vi "Set Emergency.vi"(8 "error in (no error)":errorcluster, 10 "Emergency":bool=TRUE, 11 "Elevator Controller in":refnum<class "Elevator Controller.lvclass">) -> (0 "error out":errorcluster, 3 "Elevator Controller out":refnum<class "Elevator Controller.lvclass">)   [LabVIEW 2019, in "Elevator Controller.lvlib" / "Elevator Controller.lvclass"]
uses:
  Elevator Controller.lvclass
  C:/Program Files (x86)/National Instruments/LabVIEW 2019/vi.lib/ActorFramework/Actor/Actor.lvclass
  <vilib>/ActorFramework/Actor/Actor.lvclass/Actor.ctl
  <vilib>/ActorFramework/Message Enqueuer/Message Enqueuer.lvclass/Message Enqueuer.ctl
  Elevator Controller.lvclass/Elevator Controller.ctl
  State -Enum.ctl
  Elevator Controller Messages/Set State Msg/Set State Msg.lvclass/Set State Msg.ctl
  Sim Display Console Actor/Sim Display Console Actor Messages/Write Emergency Msg/Write Emergency Msg.lvclass/Write Emergency Msg.ctl
  Sim Display Console Actor/Sim Display Console Actor Messages/Write Elevator Location Msg/Write Elevator Location Msg.lvclass/Write Elevator Location Msg.ctl
  <vilib>/ActorFramework/Message Enqueuer/Init from Existing Queue.vi
  <vilib>/ActorFramework/Message Enqueuer/Enqueue.vi
  Elevator Controller Messages/Set State Msg/Set State Msg.lvclass
  C:/Program Files (x86)/National Instruments/LabVIEW 2019/vi.lib/ActorFramework/Message/Message.lvclass
  Sim Display Console Actor/Sim Display Console Actor Messages/Write Emergency Msg/Write Emergency Msg.lvclass
  Sim Display Console Actor/Sim Display Console Actor Messages/Write Elevator Location Msg/Write Elevator Location Msg.lvclass
  <vilib>/ActorFramework/Message Priority Queue/Priority Enqueue.vi
  <vilib>/ActorFramework/Message Enqueuer/Message Enqueuer.lvclass
  <vilib>/ActorFramework/Actor/Actor.lvclass
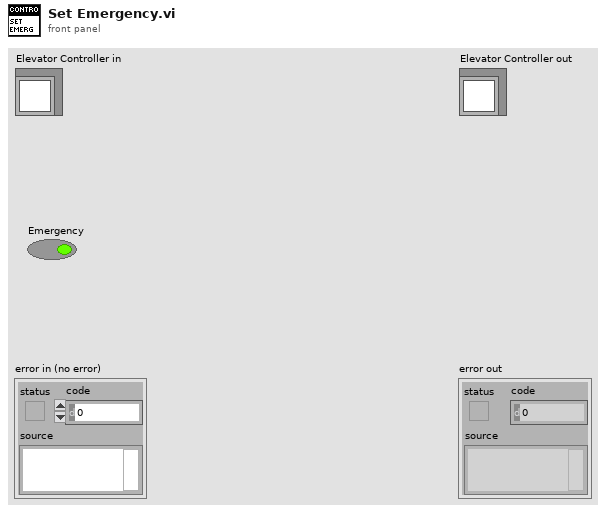
[diagram p1: front panel]
types:
  T1 = typedef "Elevator Controller.lvlib/Elevator Controller.lvclass/State -Enum.ctl" = enum16{"Initial", "Wait for First Request", "Start and Move", "Analysis", "Continue Travel", "Stop at Floor", "Open and Close Door Sequence", "No request Remaining", "Emergency Call", "Terminate Process"}
  T2 = typedef "Sim Display Console Actor.lvlib/Sim Display Console Actor.lvclass/Floors -Enum.ctl" = enum16{"1st Floor", "2nd Floor", "3rd Floor", "4th Floor"}
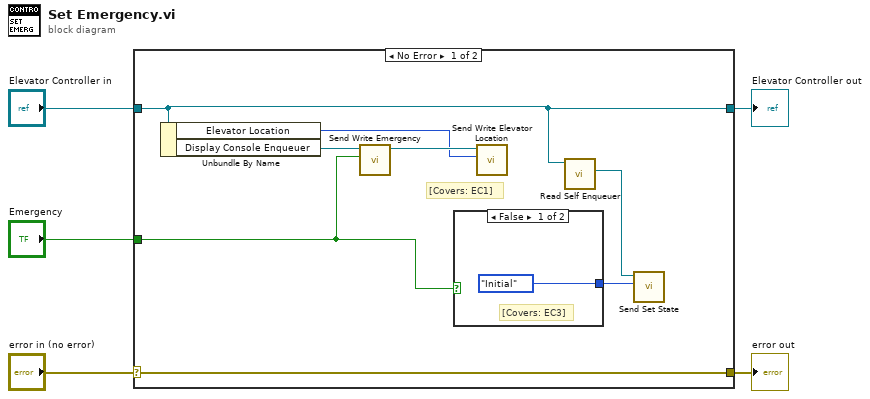
[diagram p0: block diagram]
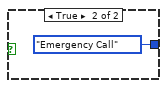
[diagram p2: hidden frame]
diagram:
  n1 = case shown="No Error" "error in (no error)" {
    selector: "error in (no error)" -> [w13 w17]
    tunnel: [w13 w17] -> w4
    tunnel: [w9 w16] -> w2
    tunnel: "Elevator Controller in" -> [w9 w16]
    tunnel: "Emergency" -> [w11 _]
    frame No Error {
      # "[Covers: EC1]"
      n2 = Unbundle By Name(w9) -> ("Elevator Location"=w6:T2, "Display Console Enqueuer"=w12:refnum<class "Message Enqueuer.lvclass">)
      n3 = call "Send Write Emergency.vi"("Emergency"=w11, "Message Enqueuer"=w12) -> ("Message Enqueuer out"=w7:refnum<class "Message Enqueuer.lvclass">)  [unwired: 8 in, 1 out]
      n4 = case shown="False" w11 {
        tunnel: [State_-Enum."Initial" ("State") State_-Enum."Emergency Call" ("State")] -> w10
        frame False {
          # "[Covers: EC3]"
        }
        frame True {
        }
      }
      n5 = call "Send Write Elevator Location.vi"("Elevator Location"=w6, "Message Enqueuer"=w7) -> ()  [unwired: 8 in, 2 out]
      n6 = call <vilib>:"Read Self Enqueuer.vi"("Actor"=w9) -> ("Self Enqueuer"=w8:refnum<class "Message Enqueuer.lvclass">)  [unwired: 10 in]
      n7 = call "Send Set State.vi"("State"=w10, "Message Enqueuer"=w8) -> ()  [unwired: 8 in, 2 out]
    }
    frame Error {
    }
  }
  "error out" <- w4
  "Elevator Controller out" <- w2
